vi "Extract State from Data.vi"(8 "error in (no error)":errorcluster, 9 "State":T4, 11 "Data In 2":T5 caption="Data In") -> (0 "error out":errorcluster, 1 "Display State Out":T4 caption="State", 2 "Waveform State Out":T1={"Show Axes"=FALSE, "Show Y=0"=FALSE, "Controls"={"Type"=enum."Sine", "Periods"=0.0, "Points"=0, "Offset"=0.0, "Amplitdue"=0.0, "Phase"=0.0, "func"=""}, "Show Current Location"=FALSE, "Current Location"=0, "dt"=0.0, "t0"=timestamp(0 s since 1904-01-01), "Format and Units"="%_3p"} caption="State", 3 "Data In":T5)   [LabVIEW 2012]
uses:
  Waveform Control.xctl
  Function Types.ctl
  FP Controls.ctl
  Controls/State.ctl
  Controls/Data.ctl
  Controls/Waveform State.ctl
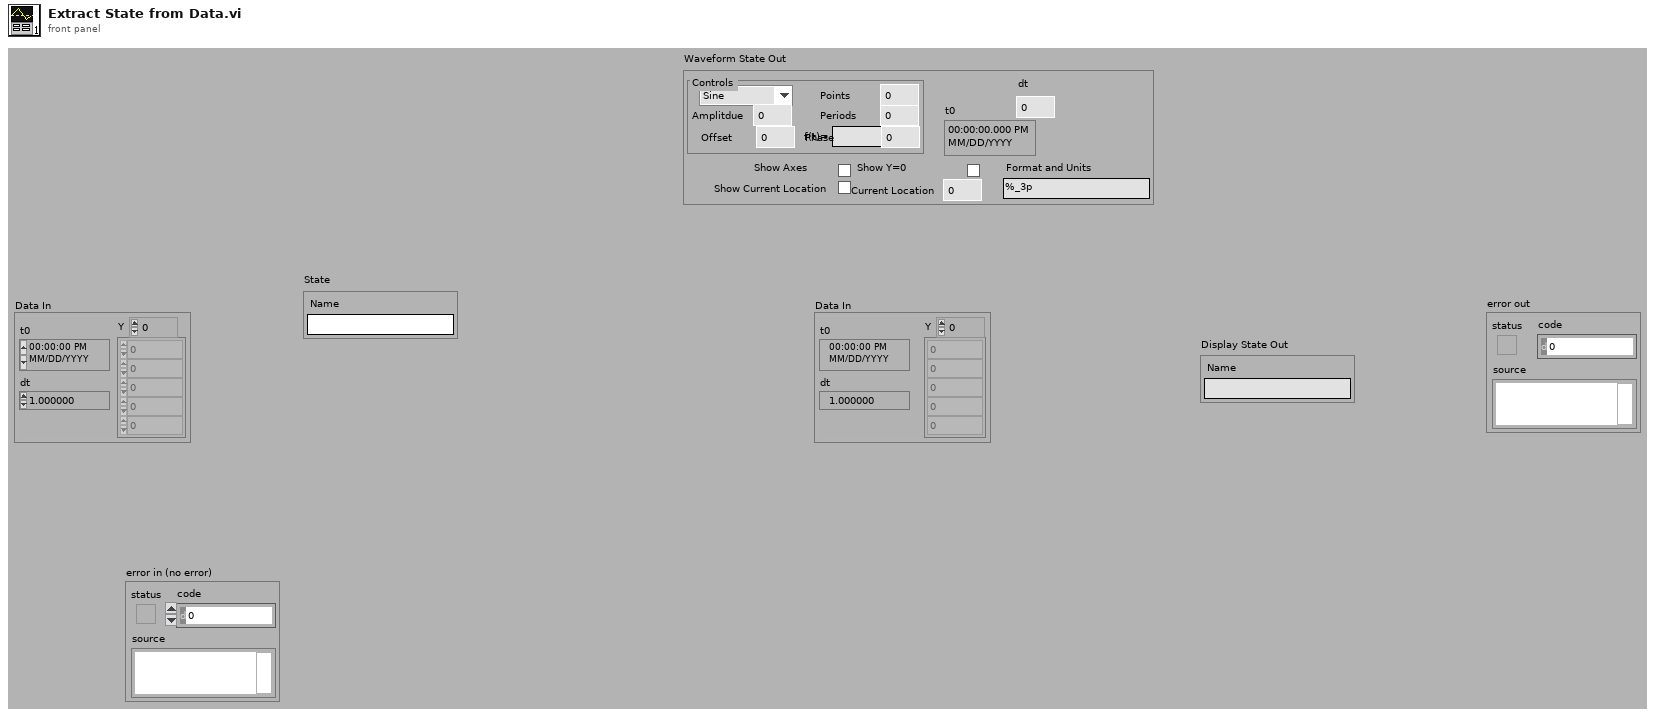
[diagram p1: front panel]
types:
  T1 = typedef "Waveform Control.xctl/Waveform State.ctl" = cluster{"Show Axes":bool, "Show Y=0":bool, "Controls":T2, "Show Current Location":bool, "Current Location":i32, "dt":dbl, "t0":timestamp, "Format and Units":string}
  T2 = typedef "Waveform Control.xctl/FP Controls.ctl" = cluster{"Type":T3, "Periods":dbl, "Points":i32, "Offset":dbl, "Amplitdue":dbl, "Phase":dbl, "func":string}
  T3 = typedef "Waveform Control.xctl/Function Types.ctl" = enum16{"Level", "Sine", "Triangle", "Ramp", "Saw Tooth", "Square", "Function"}
  T4 = typedef "Waveform Control.xctl/State.ctl" = cluster{"Name":string}
  T5 = typedef "Waveform Control.xctl/Data.ctl" = waveform(dbl)
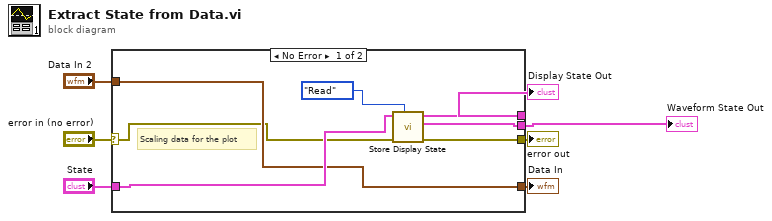
[diagram p0: block diagram]
diagram:
  n1 = case shown="No Error" "error in (no error)" {
    selector: "error in (no error)" -> [w9 w16]
    tunnel: [w14 w16] -> w7
    tunnel: [w13 _] -> w5
    tunnel: [w10 w15] -> w4
    tunnel: "Data In 2" -> [w10 w15]
    tunnel: "State" -> [w11 _]
    tunnel: [w8 _] -> w1
    frame No Error {
      # "Scaling data for the plot"
      n2 = call "Store Display State.vi"("Operation In"=enum16{"Read", "Write"}."Read" ("Operation"), "Error In (no Error) In"=w9, "State In"=w11) -> ("Error Out"=w14:errorcluster, "Waveform State Out"=w8:T1, "Display State Out"=w13:T4)  [unwired: 3 in, 3 out]
    }
    frame Error {
    }
  }
  "error out" <- w7
  "Display State Out" <- w5
  "Data In" <- w4
  "Waveform State Out" <- w1
